vi "Render.vi"(8 "error in (no error)":errorcluster, 10 "Destination":T1, 11 "Animated Texture in":refnum<class "Animated Texture.lvclass">) -> (0 "error out":errorcluster)   [LabVIEW 2015, in "Animated Texture.lvclass"]
uses:
  Animated Texture.lvclass
  Texture/Texture.lvclass
  LabSDL2/Source/Libraries/SDL2 Utility/Point (I32).ctl
  LabSDL2/Source/Libraries/SDL2 Utility/SDL2 Utility.lvlib
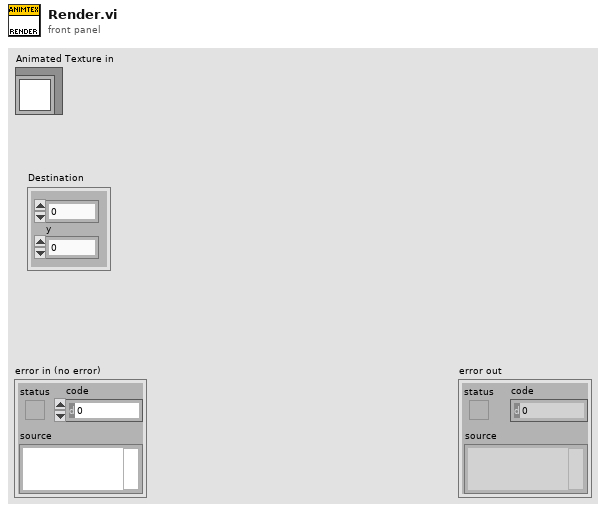
[diagram p1: front panel]
types:
  T1 = typedef "SDL2 Utility.lvlib/Point (I32).ctl" = cluster{"x":i32, "y":i32}
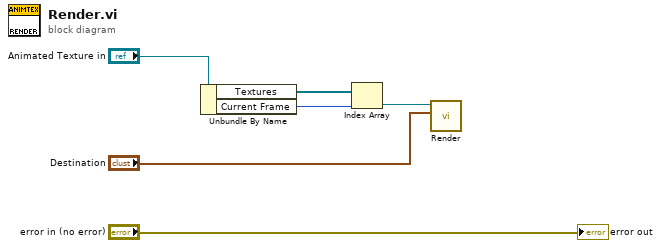
[diagram p0: block diagram]
diagram:
  n1 = Unbundle By Name("Animated Texture in") -> ("Textures"=w3:refnum<class "Texture.lvclass">[], "Current Frame"=w4:i32)
  n2 = Index Array(array=w3, index=w4) -> (element=w2:refnum<class "Texture.lvclass">)
  n3 = call-dynamic "Render.vi"("Destination"="Destination", "Texture in"=w2) -> ()  [unwired: 9 in, 1 out]
  "error out" <- "error in (no error)"
